vi "Get  Listbox click row index.vi"(8 "error in (no error)":errorcluster, 10 "Coords":T1, 11 "CtlRef Input":refnum<vi>) -> (0 "error out":errorcluster, 2 "Row":i32, 3 "CtlRef OutPut":refnum<vi>)   [LabVIEW 2020, in "John_vi_lib.lvlib"]
uses:
  John_vi_lib.lvlib
  <vilib>/Utility/miscctls.llb/LVPoint32TypeDef.ctl
  <vilib>/Utility/miscctls.llb/LVPositionTypeDef.ctl
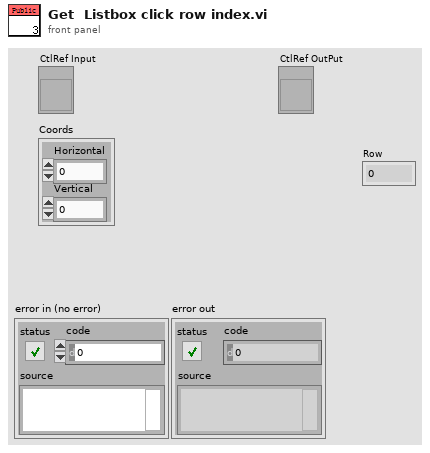
[diagram p1: front panel]
types:
  T1 = typedef "LVPoint32TypeDef.ctl" = cluster{"Horizontal":i32, "Vertical":i32}
  T2 = typedef "LVPositionTypeDef.ctl" = cluster{"Left":i32, "Top":i32}
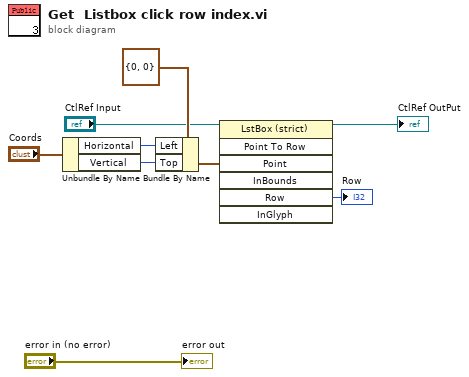
[diagram p0: block diagram]
diagram:
  n1 = Unbundle By Name("Coords") -> ("Horizontal"=w8:i32, "Vertical"=w9:i32)
  n2 = Bundle By Name(cluster=T2 {"Left"=0, "Top"=0} ("Point"), "Left"=w8, "Top"=w9) -> (w6:T2)
  n3 = invoke class="LstBox (strict)" method="Point To Row"(reference="CtlRef Input", "Point"=w6) -> (reference out=→"CtlRef OutPut":refnum<vi>, "Row"=→"Row":i32)  [unwired: 5 in, 5 out]
  "error out" <- "error in (no error)"
